vi "Write Projects.vi"(8 "error in (no error)":errorcluster, 10 "Projects":map{string, set{string}}(c390), 11 "Projects in":refnum<class "Projects.lvclass">) -> (0 "error out":errorcluster, 3 "Projects out":refnum<class "Projects.lvclass">)   [LabVIEW 2020, in "Projects.lvclass"]
uses:
  Projects.lvclass
  Projects.lvclass/Projects.ctl
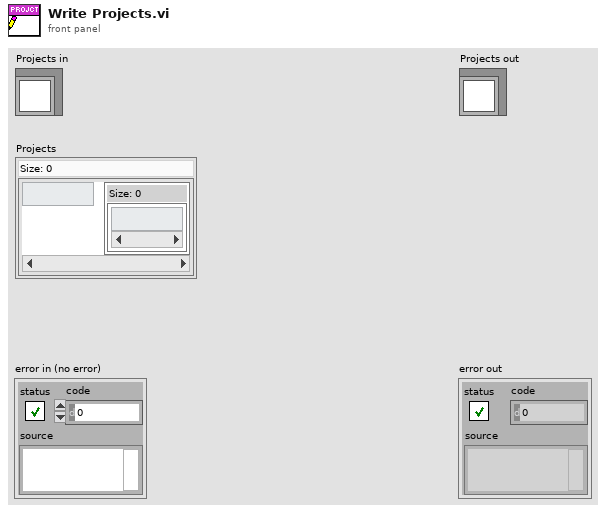
[diagram p1: front panel]
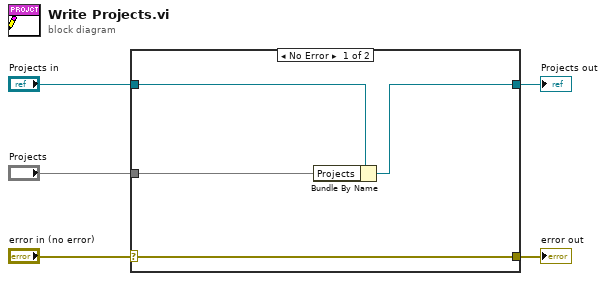
[diagram p0: block diagram]
diagram:
  n1 = case shown="No Error" "error in (no error)" {
    selector: "error in (no error)" -> [w9 w10]
    tunnel: [w9 w10] -> w4
    tunnel: [w7 w11] -> w2
    tunnel: "Projects in" -> [w8 w11]
    tunnel: "Projects" -> [w6 _]
    frame No Error {
      n2 = Bundle By Name(cluster=w8, "Projects"=w6) -> (w7:refnum<class "Projects.lvclass">)
    }
    frame Error {
    }
  }
  "error out" <- w4
  "Projects out" <- w2
